vi "ingest.ingest_run.vi"(6 "Existing Data Sources":string[](array[string]), 7 "Properties and Labels":cluster{"properties":string, "labels":string}, 8 "error in":errorcluster, 9 "Start Time":T1, 10 "Title":cluster{"Name":string, "Description":string}, 11 "Nominal Client in":refnum<class "Nominal Client.lvclass">) -> (0 "error out":errorcluster, 2 "runRid":string, 3 "Nominal Client out":refnum<class "Nominal Client.lvclass">, 4 "Response":string)   [LabVIEW 2018, in "Nominal Client.lvclass"]
doc: "Creates a run and ingests data sources to be added to the run."
uses:
  Nominal Client.lvclass
  <vilib>/JDP Science/JSONtext/LVClass Serializer/JSONtext LVClass Serializer.lvclass
  4b965f09-dc68-4d5e-a5c1-32d476accfd4.vi
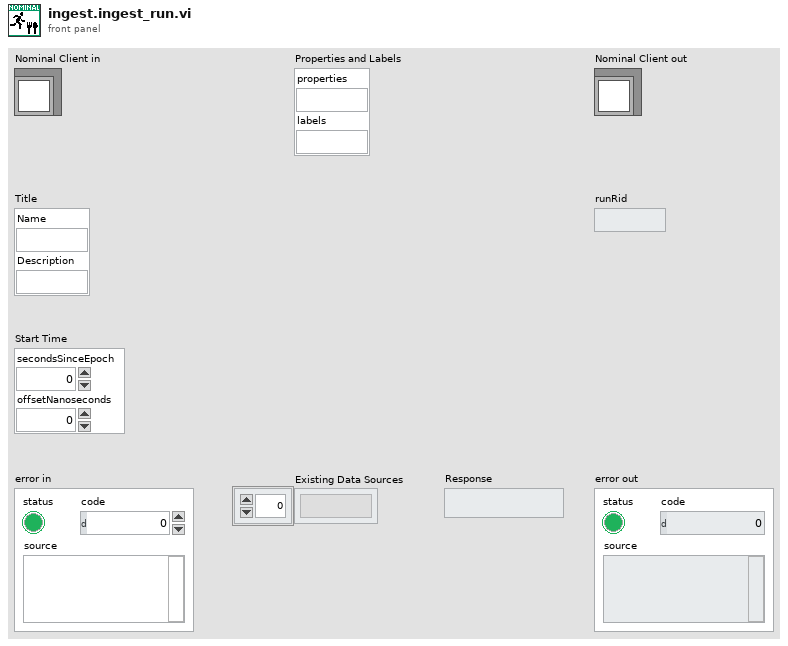
[diagram p1: front panel]
types:
  T1 = cluster{"secondsSinceEpoch":i32, "offsetNanoseconds":i32}
  T2 = cluster{"title":string, "description":string, "startTime":cluster{"secondsSinceEpoch":i32, "offsetNanoseconds":i32}, "properties":string, "labels":string, "dataSource":cluster{"Existing Data Source":cluster{"type":string, "existingDataSource":string}[]}}
  T3 = cluster{"type":string, "Existing Data Source":string}
  T4 = cluster{cluster{"type":string, "Existing Data Source":string}[]}
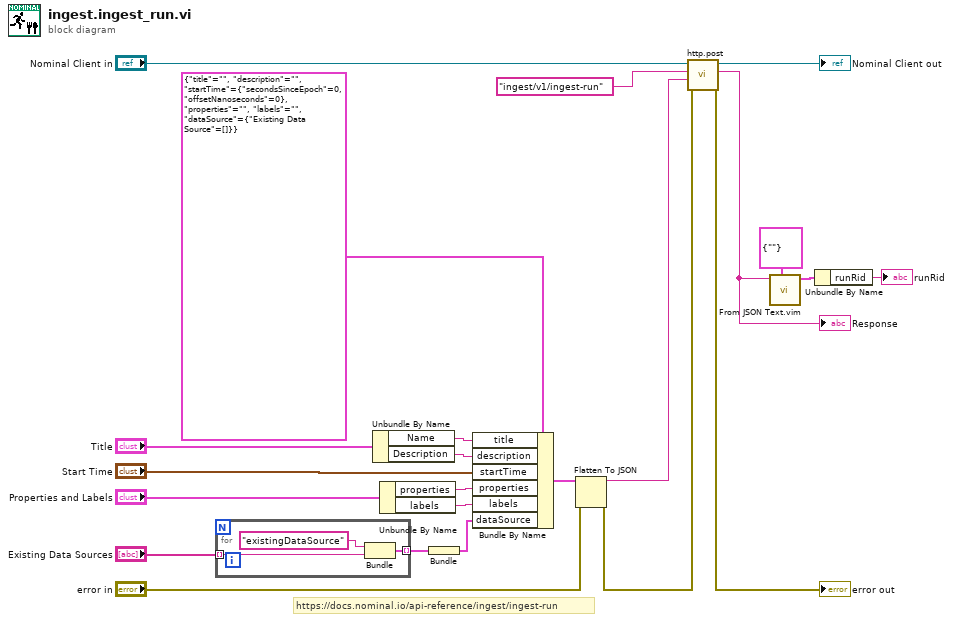
[diagram p0: block diagram]
diagram:
  # "https://docs.nominal.io/api-reference/ingest/ingest-run"
  n1 = for {
    tunnel: "Existing Data Sources" -> [w26] mode=indexing
    tunnel: [w24] -> w5 mode=indexing
    n2 = Bundle("type"="existingDataSource", "Existing Data Source"=w26) -> (w24:T3)  [unwired: 1 in]
  }
  n3 = Unbundle By Name("Title") -> ("Name"=w9:string, "Description"=w8:string)
  n4 = Unbundle By Name("Properties and Labels") -> ("properties"=w2:string, "labels"=w1:string)
  n5 = Bundle(w5) -> (w4:T4)  [unwired: 1 in]
  n6 = Bundle By Name(cluster=T2 {"title"="", "description"="", "startTime"={"secondsSinceEpoch"=0, "offsetNanoseconds"=0}, "properties"="", "labels"="", "dataSource"={"Existing Data Source"=[]}}, "title"=w9, "description"=w8, "startTime"="Start Time", "properties"=w2, "labels"=w1, "dataSource"=w4) -> (w11:T2)
  n7 = Flatten To JSON(anything=w11, error in (no error)="error in") -> (JSON string=w19:string, 11:w18:errorcluster)  [unwired: 1 in]
  n8 = call "http.post.vi"("error in"=w18, "Request body"=w19, "Path"="ingest/v1/ingest-run", "Nominal Client in"="Nominal Client in") -> ("error out"=→"error out":errorcluster, "Response"=w15:string, "Nominal Client out"=→"Nominal Client out":refnum<class "Nominal Client.lvclass">)  [unwired: 4 in, 1 out]
  "Response" <- w15
  n9 = call "From JSON Text.vim"("Data Type and Default Value"=cluster{"runRid":string} {"runRid"=""} ("Information"), "JSON"=w15) -> ("Data out"=w14:cluster{"runRid":string})  [unwired: 8 in, 1 out]
  n10 = Unbundle By Name(w14) -> ("runRid"=→"runRid":string)
